vi "1710_模拟量输入.vi"() -> ()   [LabVIEW 2015]
uses:
  <userlib>/DAQNavi Polymorphic VI/create/DAQNavi Create Channel(AI-Voltage).vi
  <userlib>/DAQNavi Polymorphic VI/read/DAQNavi Read (Analog DBL 1Chan 1Samp).vi
panel:
  out "波形图表":dbl[](graph)
  out "data":dbl
  out "error out":errorcluster
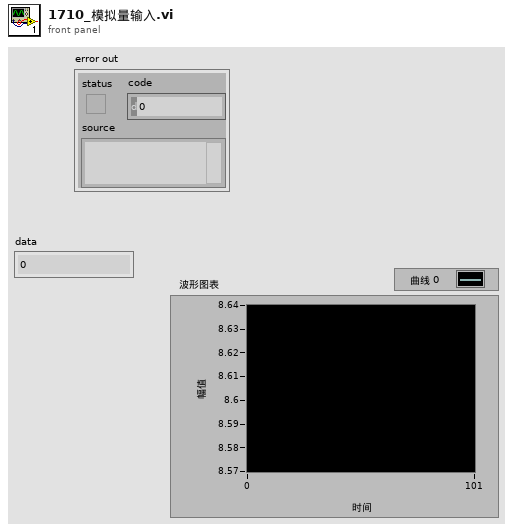
[diagram p1: front panel]
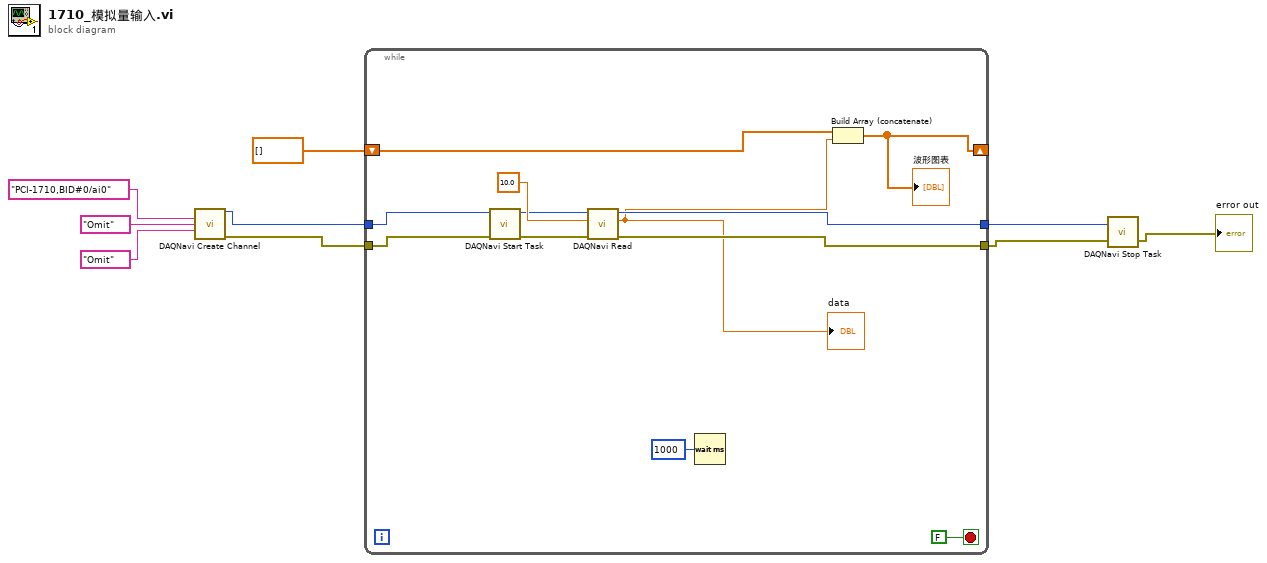
[diagram p0: block diagram]
diagram:
  n1 = call-poly <userlib>:"DAQNavi Create Channel.vi"("physical channels"="PCI-1710,BID#0/ai0", "signal type"="Omit", "value range"="Omit") -> ("task out"=w6:i32, "error out"=w5:errorcluster)  [unwired: 11 in]
  n2 = while {
    tunnel: w6 -> [w20]
    tunnel: [w16] -> w4
    tunnel: w5 -> [w19]
    tunnel: [w15] -> w3
    shift-right: [w10] -> _
    shift-left: dbl[] [] -> [w13]
    stop <- FALSE stop-if-true
    n3 = call <userlib>:"DAQNavi Start Task.vi"("error in (no error)"=w19, "task in"=w20) -> ("error out"=w18:errorcluster, "task out"=w17:i32)  [unwired: 8 in]
    n4 = call-poly <userlib>:"DAQNavi Read.vi"("error in (no error)"=w18, "timeout"=10.0, "task in"=w17) -> ("error out"=w15:errorcluster, "data"=w12:dbl, "task out"=w16:i32)  [unwired: 6 in]
    "data" <- w12
    n5 = Wait (ms)(milliseconds to wait=u32 1000 ("等待时间（毫秒）")) -> ()  [unwired: 1 out]
    n6 = Build Array (concatenate)(w13, w12) -> (w10:dbl[])
    "波形图表" <- w10
  }
  n7 = call <userlib>:"DAQNavi Stop Task.vi"("error in (no error)"=w3, "task in"=w4) -> ("error out"=→"error out":errorcluster)  [unwired: 1 out]
